vi "CCUP.vi"(3 "Device Category IN:":string(combo)="ATLAS18SS" caption="Device Category:", 4 "Batch No.:":string, 5 "Sensor Serial No.:":string, 6 "DB Serial No.:":string) -> (0 "Done!":bool)   [LabVIEW 2019]
doc: "Performs CV measurements according to ATLAS ITk Quality Control Specifications."
uses:
  general_VIs/globals/QC_RunInformation.vi
  general_VIs/globals/QC_MeasurementSetup.vi
  InstrControl/InstrumentSetup.vi
  InstrControl/Switching/Switching.lvclass
  InstrControl/SupplyControl/SupplyControl.lvclass
  InstrControl/LCRControl/LCRControl.lvclass
  InstrControl/ArduinoControl/ArduinoControl.lvclass
  <vilib>/Analysis/NI_AALBase.lvlib
  InstrControl/InstrControl.lvclass
panel:
  out "positive ramp?":bool
  out "Measured Capacitance [pF]":dbl
  in  "Continue":bool
  out "RH":dbl[](array[numeric]) caption="RH [%]" format="%#.2f"
  out "Temp.":dbl[](array[numeric]) caption="Temp. [°C]" format="%#.2f"
  in  "Measurement Configurations":bool
  in  "Frequency [Hz] Setup":i32=500 caption="Frequency [Hz]" format="%#.3p"
  in  "step interval [s] IN":i32=5 caption="step interval [s]"
  in  "step [V] IN":dbl=10.0 caption="step [V]" format="%.1f"
  in  "Final volts [V] IN":dbl=-500.0 caption="Final volts [V]"
  in  "Initial volts [V] IN":dbl caption="Initial volts [V]"
  in  "quit (no save)":bool
  in  "Quit & Save":bool
  out "Bias On/Off:":bool
  in  "Switching":string(combo)="Pickering Matrix"
  in  "Temperature":enum16{"Read Arduino", "Enter manually"}(ring)
  in  "LCR Meter":string(combo)="WayneKerr 6440B"
  in  "CV Supply":string(combo)="Keithley 2410"
  out "Initiated:":string
  in  "User:":string(combo)="Christoph"
  in  "Structure Name:":string
  # "Strip Sensor QC: Coupling Capacitance"
  # "DUT Description"
  # "Measurement Configuration"
  # "Hardware"
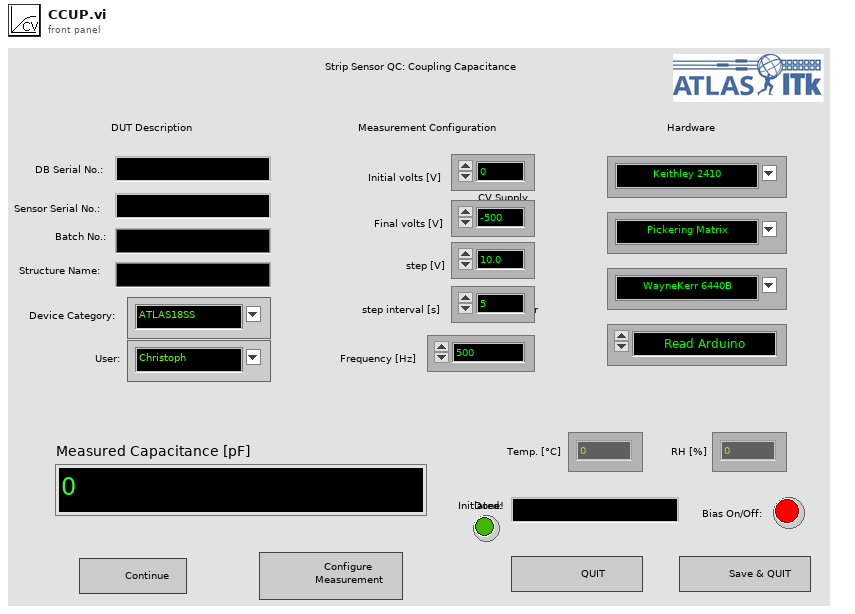
[diagram p1: front panel]
types:
  T1 = enum8{"Enabled", "Disabled", "Disabled and Grayed Out"}
  T2 = enum16{"Supply", "LCR", "Multimeter", "Switching"}
  T3 = enum16{"Reset", "Read Array", "Read Element", "Write Element", "Write Array", "Add Element", "Add Array"}
  T4 = enum16{"Reset", "Ground", "Striptest Bias", "Striptest SMU", "Striptest LCR", "IV", "CV", "Interstrip Cap", "Interstrip Res"}
  T5 = enum16{"Reset", "Ground", "Striptest Bias", "Striptest SMU", "Striptest LCR", "IV", "CV", "Interstrip Cap", "Interstrip Res", "PTP", "Implant Resistance", "Metal Resistance", "Coupling Capacitance"}
  T6 = cluster{"Supply":refnum<class "SupplyControl.lvclass">, "LCR":refnum<class "LCRControl.lvclass">, "Initial Voltage [V]":dbl, "Final Voltage [V]":dbl, "Step Size [V]":dbl, "Step Interval [s]":i32, "Number Of Steps":u32, "AC frequency [Hz]":i32, "RC Configuration":u16, "AC amplitude [V]":dbl, "Ramp down steps [V]":dbl, "Ramp down Interval [s]":i32, "Set Current Limit?":bool, "Current Limit [µA]":dbl, "Temperature Readout":enum16{"Read Arduino", "Enter manually"}, "Arduino":refnum<class "ArduinoControl.lvclass">, "Supply Name":string, "LCR Name":string, "V_depletion Limit [V]":dbl, "Switching":refnum<class "Switching.lvclass">, "Matrix used?":bool, "Matrix X Channels":cluster{"Bias Supply / SMU LO":i32, "Bias Supply / SMU HI":i32, "CV Box LO":i32, "CV Box HI":i32, "CV Box LO IN":i32, "CV Box HI IN":i32, "Volt meter LO":i32, "Volt meter HI":i32, "Mux1 C1":i32, "Mux1 C2":i32, "Mux2 C1":i32, "Mux2 C2":i32}, "Structure Name":string}
  T7 = cluster{"Sensor Serial No.:":string, "Wafer Serial No.:":string, "Batch:":string, "Manufacturer:":string, "Device Category:":string, "Database Serial No.:":string, "Date Initiated:":string, "Time Initiated:":string, "Test":string, "Instruments used:":string, "Probeplan used:":string, "End of Run comment:":string, "User:":string}
  T8 = cluster{"Institute":string, "Manufacturers":string[], "Devices":string[], "Serialnumbers Lookup DB":string, "Data directory":string, "Backup & screenshot directory":string, "List of known users":string[], "Measurement switch not used":bool, "Measurement Switch":string, "DUT Switch":string}
  T9 = cluster{"RC Configuration":u16, "AC amplitude [V]":dbl, "AC frequency [Hz]":i32, "WK6440B":refnum<class "WK6440B.lvclass">}
  T10 = cluster{"VISA address":refnum<visa-resource-name>, "T sensor":enum16{"SHT", "DS"}, "Arduino":refnum<class "ArduinoControl.lvclass">}
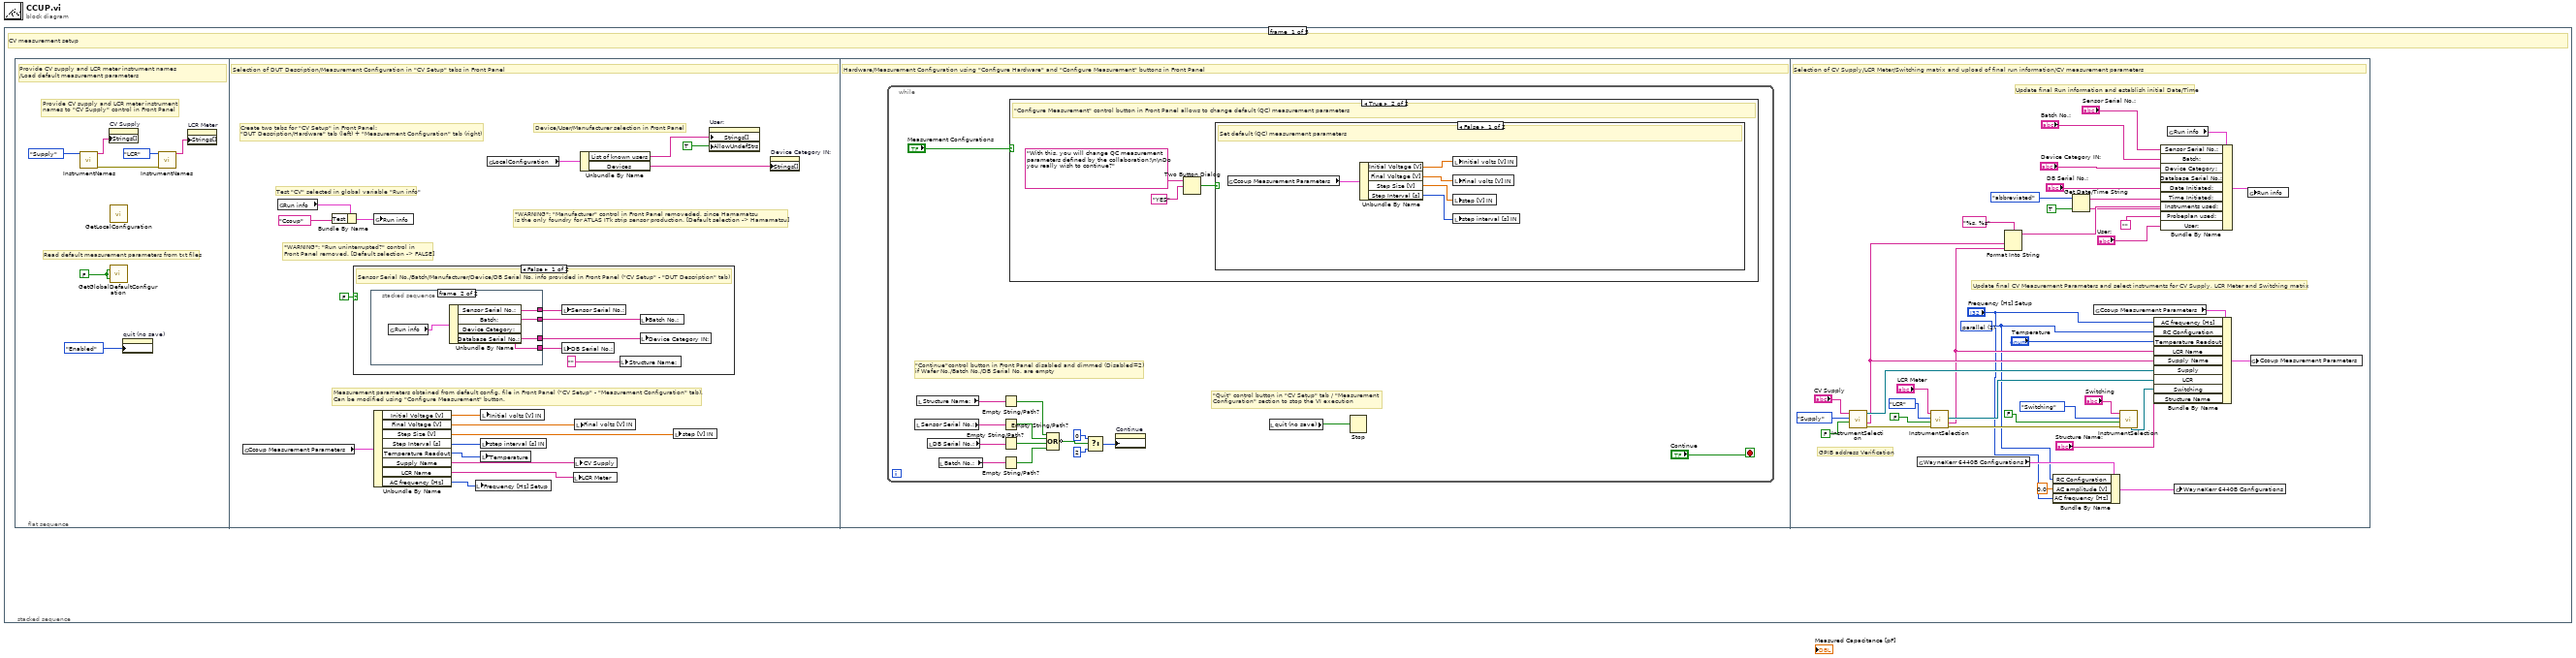
[diagram p0: block diagram]
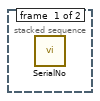
[diagram p2: hidden frame]
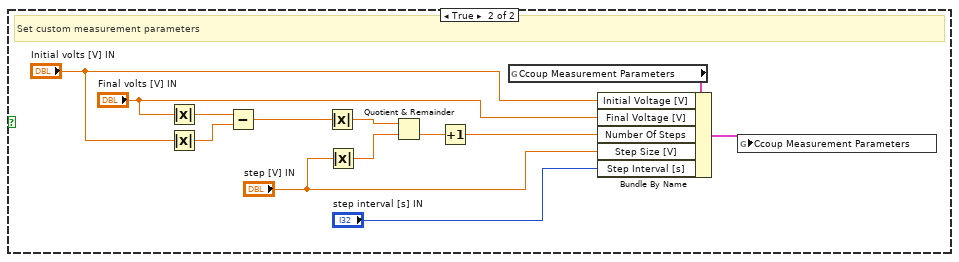
[diagram p5: hidden frame]
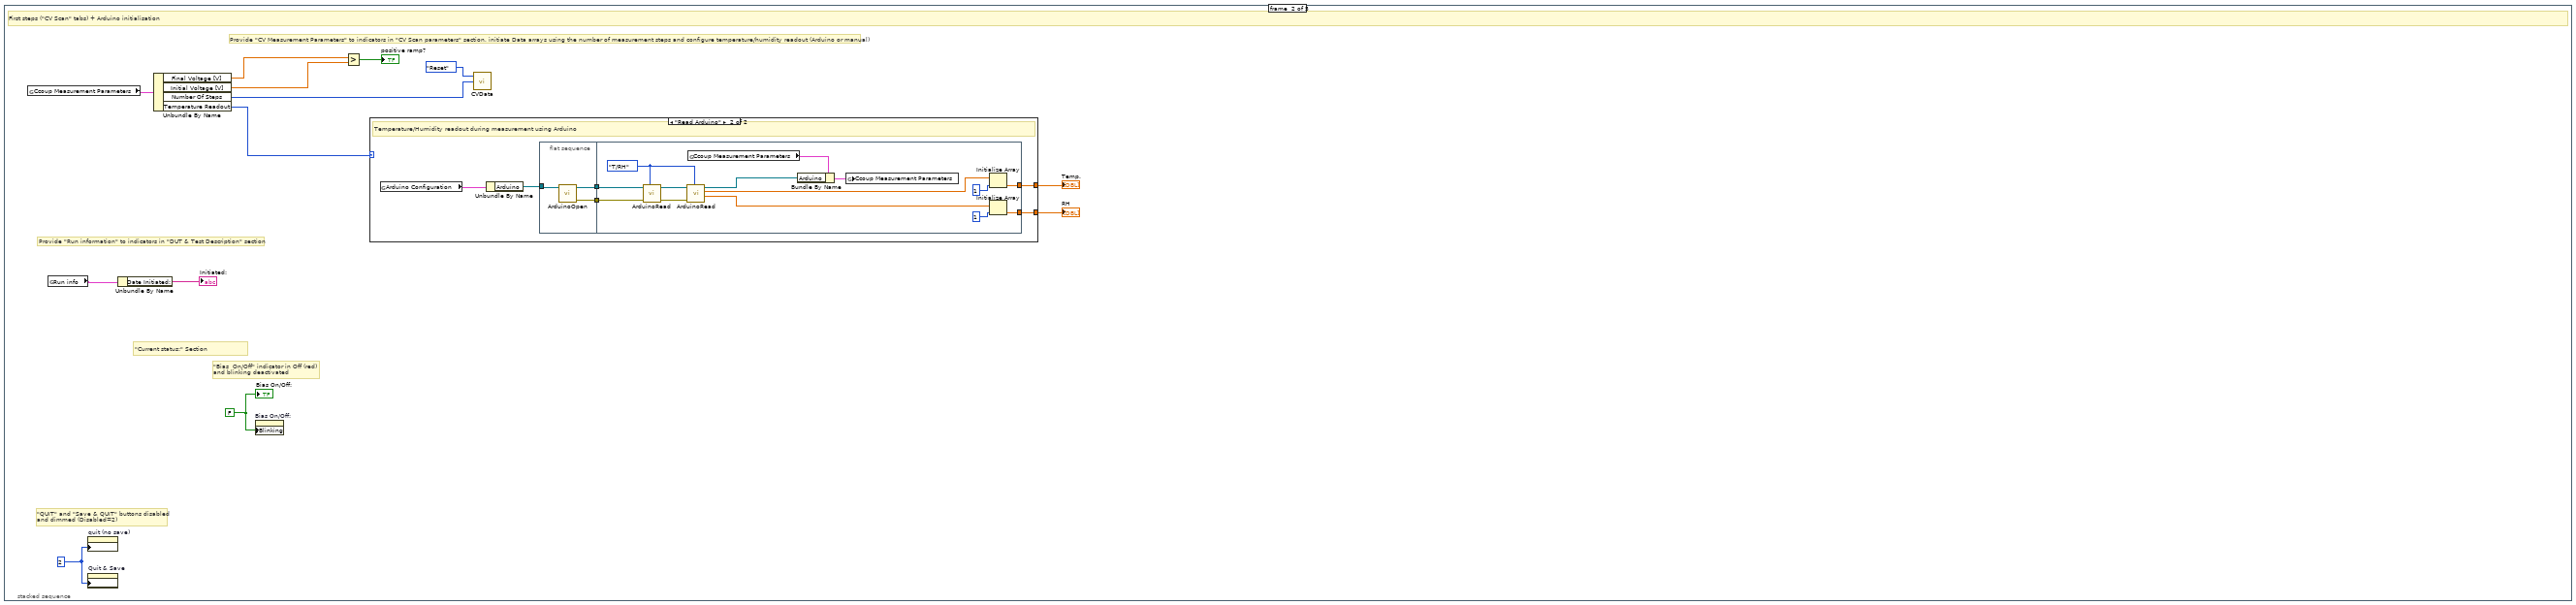
[diagram p6: hidden frame]
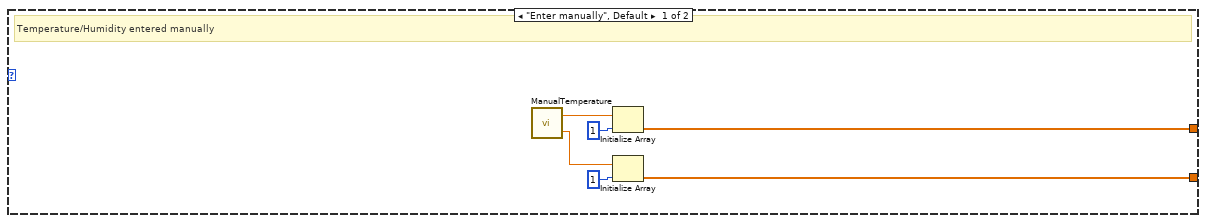
[diagram p7: hidden frame]
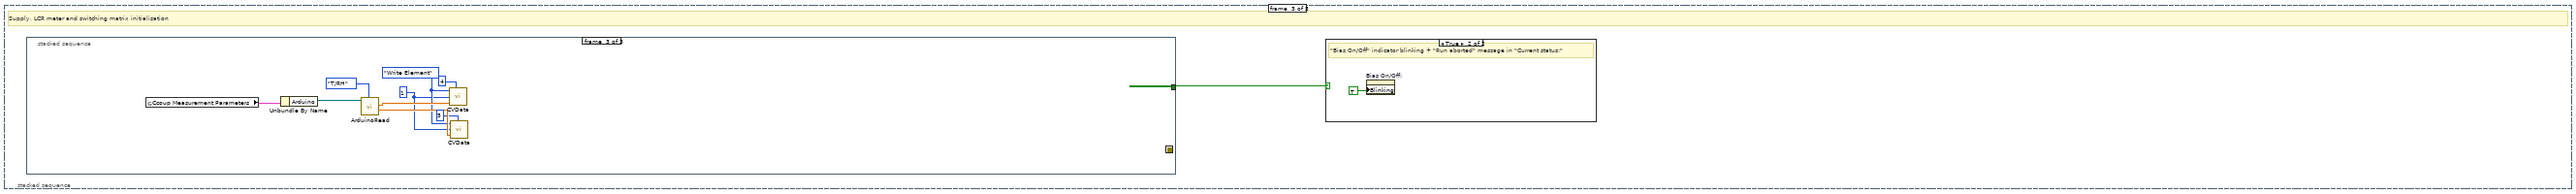
[diagram p8: hidden frame]
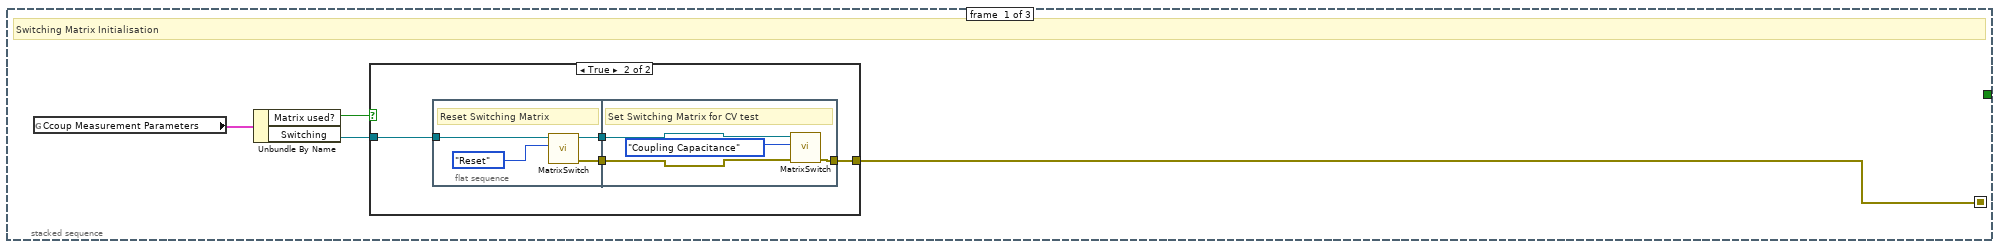
[diagram p9: hidden frame]
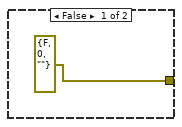
[diagram p10: hidden frame]
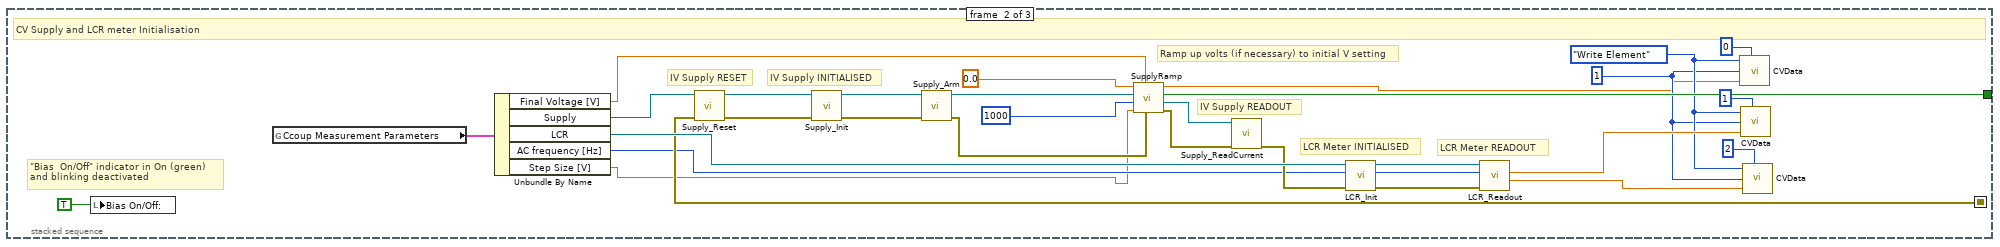
[diagram p11: hidden frame]
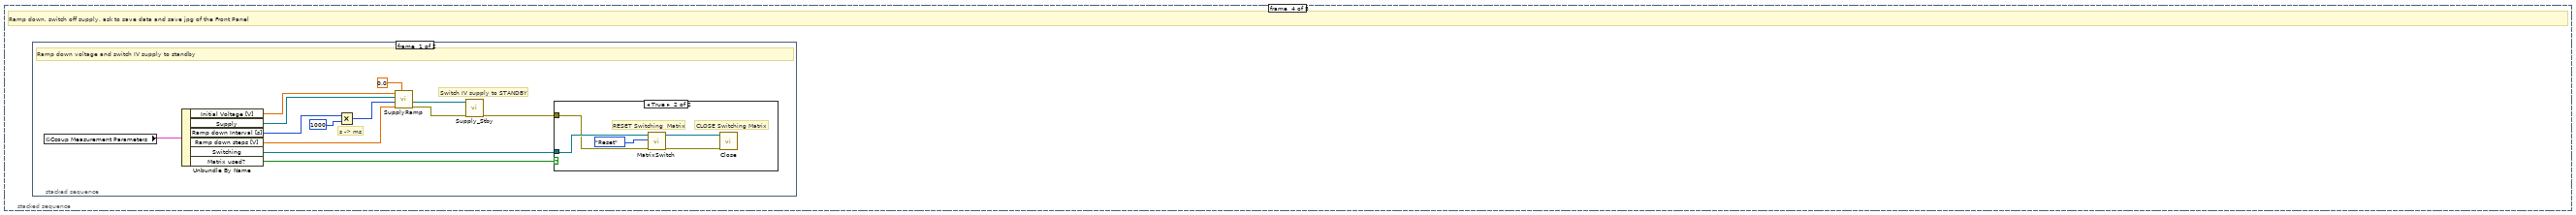
[diagram p13: hidden frame]
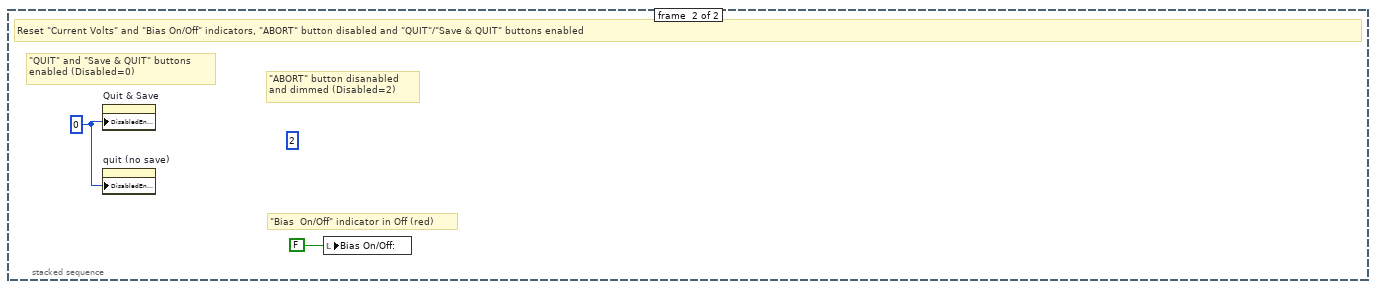
[diagram p15: hidden frame]
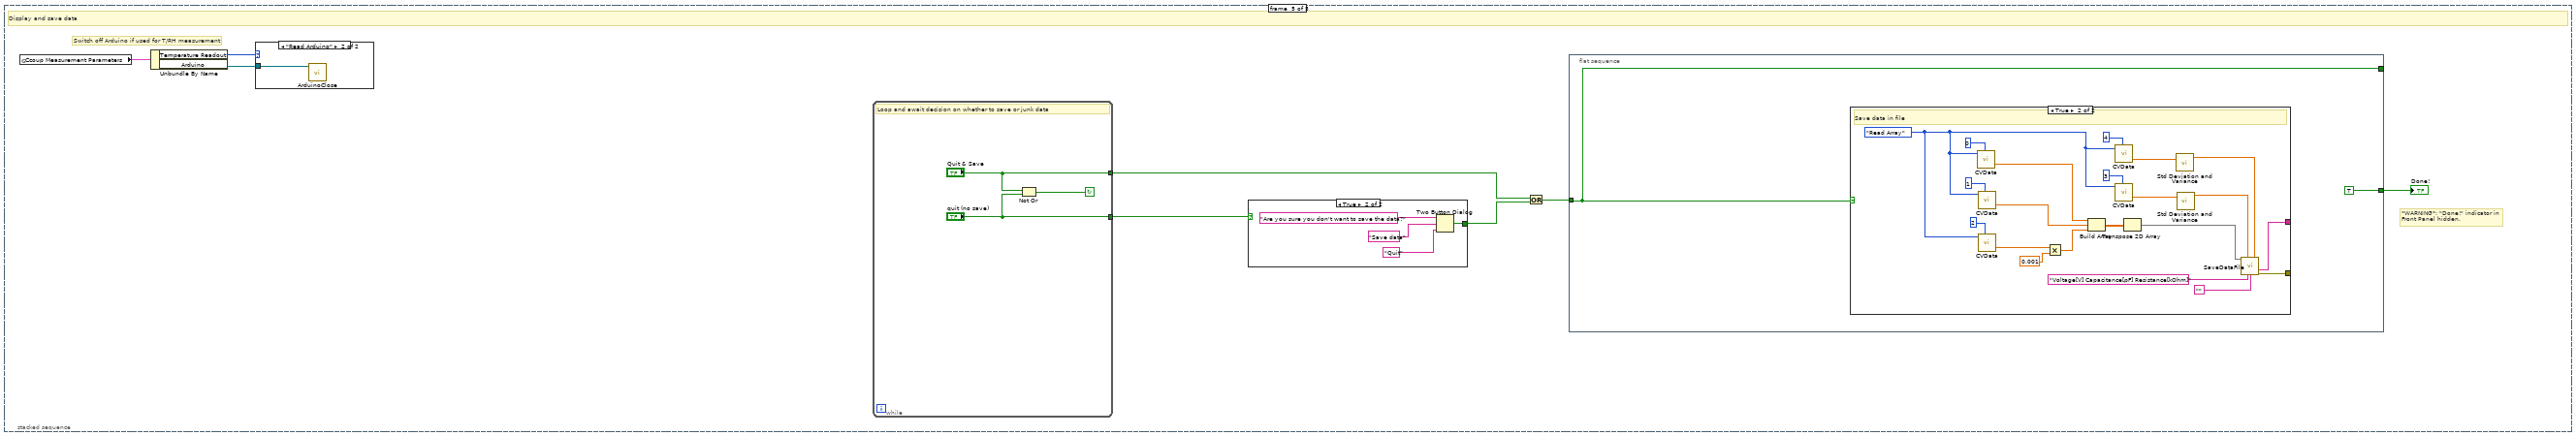
[diagram p16: hidden frame]
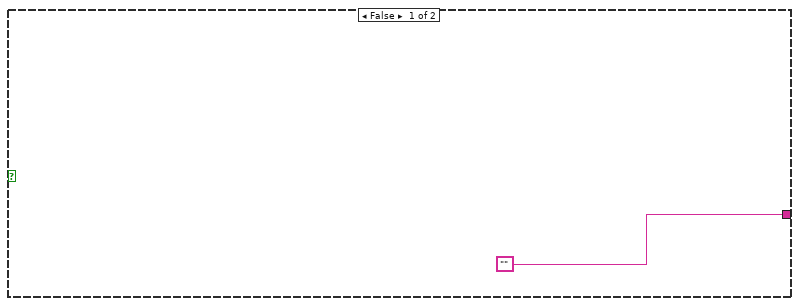
[diagram p17: hidden frame]
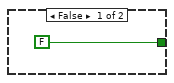
[diagram p19: hidden frame]
diagram:
  n1 = stacked-sequence {
    frame #0 {
      # "CV measurement setup"
      n2 = flat-sequence {
        frame #0 {
          w7 = FALSE
          # "Read default measurement parameters from txt files"
          # "Provide CV supply and LCR meter instrument \nnames to \"CV Supply\" control in Front Panel"
          # "Provide CV supply and LCR meter instrument names\n/Load default measurement parameters"
          n3 = call "InstrumentNames.vi"("Instrument type"=T2."Supply") -> ("error out"=w2:errorcluster, "Instrument names"=w4:string[])  [unwired: 9 in]
          n4 = property on="CV Supply" class="CmbBox"("Strings[]"=w4) -> ()  [unwired: 2 in, 2 out]
          n5 = call "GetGlobalDefaultConfiguration.vi"("DO NOT override instruments"=w7, "Read defaults?"=w7) -> ()  [unwired: 1 in, 1 out]
          n6 = call "GetLocalConfiguration.vi"() -> ()  [unwired: 3 in, 1 out]
          n7 = property on="quit (no save)" class="Bool (strict)"("DisabledEnum"=T1."Enabled" ("Disabled")) -> ()  [unwired: 2 in, 2 out]
          n8 = call "InstrumentNames.vi"("error in (no error)"=w2, "Instrument type"=T2."LCR") -> ("Instrument names"=w3:string[])  [unwired: 8 in, 1 out]
          n9 = property on="LCR Meter" class="CmbBox"("Strings[]"=w3) -> ()  [unwired: 2 in, 2 out]
        }
        frame #1 {
          # "Measurement parameters obtained from default config. file in Front Panel (\"CV Setup\" - \"Measurement Configuration\" tab).\nCan be modified using \"Configure Measurement\" button."
          # "*WARNING*: \"Run uninterrupted?\" control in \nFront Panel removed. [Default selection -> FALSE]"
          # "*WARNING*: \"Manufacturer\" control in Front Panel removeded, since Hamamatsu \nis the only foundry for ATLAS ITk strip sensor production. [Default selection -> Hamamatsu]"
          # "Test \"CV\" selected in global variable \"Run info\""
          # "Device/User/Manufacturer selection in Front Panel"
          # "Create two tabs for \"CV Setup\" in Front Panel:\n\"DUT Description/Hardware\" tab (left) + \"Measurement Configuration\" tab (right)"
          # "Selection of DUT Description/Measurement Configuration in \"CV Setup\" tabs in Front Panel"
          n10 = global read "QC_MeasurementSetup.vi" "Ccoup Measurement Parameters"() -> (w22:T6)
          n11 = global read "QC_RunInformation.vi" "Run info"() -> (w15:T7)
          n12 = Bundle By Name(cluster=w15, "Test"="Ccoup") -> (w16:T7)
          n13 = case shown="False" FALSE {
            frame False {
              # "Sensor Serial No./Batch/Manufacturer/Device/DB Serial No. info provided in Front Panel (\"CV Setup\" - \"DUT Description\" tab)"
              n14 = stacked-sequence {
                tunnel: [_ w34] -> w28
                tunnel: [_ w33] -> w27
                tunnel: [_ w32] -> w29
                tunnel: [_ w30] -> w26
                frame #0 {
                  n15 = call "SerialNo.vi"() -> ()  [unwired: 5 in, 1 out]
                }
                frame #1 {
                  n16 = global read "QC_RunInformation.vi" "Run info"() -> (w31:T7)
                  n17 = Unbundle By Name(w31) -> ("Sensor Serial No.:"=w34:string, "Batch:"=w33:string, "Device Category:"=w32:string, "Database Serial No.:"=w30:string)
                }
              }
              n18 = local write "Sensor Serial No.:"(w28) -> ()
              n19 = local write "DB Serial No.:"(w26) -> ()
              n20 = local write "Structure Name:"("" ("Structure Name:")) -> ()
              n21 = local write "Batch No.:"(w27) -> ()
              n22 = local write "Device Category IN:"(w29) -> ()
            }
            frame True {
            }
          }
          n23 = global write "QC_RunInformation.vi" "Run info"(w16) -> ()
          n24 = Unbundle By Name(w22) -> ("Initial Voltage [V]"=w11:dbl, "Final Voltage [V]"=w12:dbl, "Step Size [V]"=w13:dbl, "Step Interval [s]"=w14:i32, "Temperature Readout"=w24:enum16{"Read Arduino", "Enter manually"}, "Supply Name"=w23:string, "LCR Name"=w18:string, "AC frequency [Hz]"=w17:i32)
          n25 = local write "Frequency [Hz] Setup"(w17) -> ()
          n26 = local write "step interval [s] IN"(w14) -> ()
          n27 = local write "Temperature"(w24) -> ()
          n28 = local write "Initial volts [V] IN"(w11) -> ()
          n29 = global read "QC_RunInformation.vi" "LocalConfiguration"() -> (w21:T8)
          n30 = local write "LCR Meter"(w18) -> ()
          n31 = local write "CV Supply"(w23) -> ()
          n32 = local write "Final volts [V] IN"(w12) -> ()
          n33 = Unbundle By Name(w21) -> ("List of known users"=w20:string[], "Devices"=w10:string[])
          n34 = local write "step [V] IN"(w13) -> ()
          n35 = property on="User:" class="CmbBox"("Strings[]"=w20, "AllowUndefStrs"=TRUE) -> ()  [unwired: 2 in, 2 out]
          n36 = property on="Device Category IN:" class="CmbBox"("Strings[]"=w10) -> ()  [unwired: 2 in, 2 out]
        }
        frame #2 {
          # "Hardware/Measurement Configuration using \"Configure Hardware\" and \"Configure Measurement\" buttons in Front Panel"
          n37 = while {
            stop <- "Continue" stop-if-true
            # "\"Continue\"control button in Front Panel disabled and dimmed (Disabled=2) \nif Wafer No./Batch No./DB Serial No. are empty"
            # "\"Quit\" control button in \"CV Setup\" tab / \"Measurement \nConfiguration\" section to stop the VI execution"
            n38 = local read "Sensor Serial No.:"() -> (w49:string)
            n39 = local read "Structure Name:"() -> (w36:string)
            n40 = local read "DB Serial No.:"() -> (w48:string)
            n41 = local read "Batch No.:"() -> (w41:string)
            n42 = Empty String/Path?(string/path=w36) -> (empty?=w35:bool)
            n43 = Empty String/Path?(string/path=w49) -> (empty?=w46:bool)
            n44 = Empty String/Path?(string/path=w48) -> (empty?=w47:bool)
            n45 = Empty String/Path?(string/path=w41) -> (empty?=w40:bool)
            n46 = case shown="True" "Measurement Configurations" {
              frame False {
              }
              frame True {
                # "\"Configure Measurement\" control button in Front Panel allows to change default (QC) measurement parameters"
                n47 = Two Button Dialog(message="With this, you will change QC measurement parameters defined by the collaboration!\n\nDo you really wish to continue?", 2:"YES") -> (T button?=w50:bool)  [unwired: 1 in]
                n48 = case shown="False" w50 {
                  frame False {
                    # "Set default (QC) measurement parameters"
                    n49 = global read "QC_MeasurementSetup.vi" "Ccoup Measurement Parameters"() -> (w57:T6)
                    n50 = Unbundle By Name(w57) -> ("Initial Voltage [V]"=w54:dbl, "Final Voltage [V]"=w53:dbl, "Step Size [V]"=w55:dbl, "Step Interval [s]"=w56:i32)
                    n51 = local write "Initial volts [V] IN"(w54) -> ()
                    n52 = local write "Final volts [V] IN"(w53) -> ()
                    n53 = local write "step [V] IN"(w55) -> ()
                    n54 = local write "step interval [s] IN"(w56) -> ()
                  }
                  frame True {
                    # "Set custom measurement parameters"
                    n55 = Absolute Value(x="Final volts [V] IN") -> (abs(x)=w64:dbl)
                    n56 = Absolute Value(x="Initial volts [V] IN") -> (abs(x)=w65:dbl)
                    n57 = Subtract(x=w64, y=w65) -> (x-y=w68:dbl)
                    n58 = Absolute Value(x=w68) -> (abs(x)=w66:dbl)
                    n59 = Absolute Value(x="step [V] IN") -> (abs(x)=w67:dbl)
                    n60 = Quotient & Remainder(x=w66, y=w67) -> (floor(x/y)=w63:dbl)  [unwired: 1 out]
                    n61 = Increment(x=w63) -> (x+1=w59:dbl)
                    n62 = global read "QC_MeasurementSetup.vi" "Ccoup Measurement Parameters"() -> (w70:T6)
                    n63 = Bundle By Name(cluster=w70, "Initial Voltage [V]"="Initial volts [V] IN", "Final Voltage [V]"="Final volts [V] IN", "Number Of Steps"=w59, "Step Size [V]"="step [V] IN", "Step Interval [s]"="step interval [s] IN") -> (w69:T6)
                    n64 = global write "QC_MeasurementSetup.vi" "Ccoup Measurement Parameters"(w69) -> ()
                  }
                }
              }
            }
            n65 = Compound Arithmetic op=OR(w35, w46, w47, w40) -> (invert w45:bool)
            n66 = Select(t=0, s=w45, f=2) -> (s? t:f=w42:i32)
            n67 = property on="Continue" class="Bool"("DisabledEnum"=w42) -> ()  [unwired: 2 in, 2 out]
            n68 = local read "quit (no save)"() -> (w38:bool)
            n69 = Stop(stop? (T)=w38) -> ()
          }
        }
        frame #3 {
          w72 = u16 1 items=["serial", "parallel"] ("RC Configuration")
          # "Update final Run information and establish initial Date/Time"
          # "Update final CV Measurement Parameters and select instruments for CV Supply, LCR Meter and Switching matrix"
          # "GPIB address Verification"
          # "Selection of CV Supply/LCR Meter/Switching matrix and upload of final run information/CV measurement parameters"
          n70 = call "InstrumentSelection.vi"("Verify GPIB address"=FALSE, "Instrument type"=T2."Supply", "Instrument name IN"="CV Supply") -> ("error out"=w95:errorcluster, "Instrument name OUT"=w78:string, "Supply"=w94:refnum<class "SupplyControl.lvclass">)  [unwired: 3 in, 3 out]
          n71 = global read "InstrumentSetup.vi" "WayneKerr 6440B Configurations"() -> (w74:T9)
          n72 = call "InstrumentSelection.vi"("error in (no error)"=w95, "Verify GPIB address"=FALSE, "Instrument type"=T2."LCR", "Instrument name IN"="LCR Meter") -> ("error out"=w91:errorcluster, "Instrument name OUT"=w77:string, "LCR"=w93:refnum<class "LCRControl.lvclass">)  [unwired: 2 in, 3 out]
          n73 = Format Into String(format string="%s, %s", w78, w77) -> (resulting string=w98:string)  [unwired: 2 in, 1 out]
          n74 = Bundle By Name(cluster=w74, "RC Configuration"=w72, "AC amplitude [V]"=0.0, "AC frequency [Hz]"="Frequency [Hz] Setup") -> (w75:T9)
          n75 = Get Date/Time String(date format (0)=enum16{"short", "long", "abbreviated"}."abbreviated", want seconds? (F)=TRUE) -> (date string=w86:string, time string=w85:string)  [unwired: 1 in]
          n76 = global read "QC_MeasurementSetup.vi" "Ccoup Measurement Parameters"() -> (w108:T6)
          n77 = call "InstrumentSelection.vi"("error in (no error)"=w91, "Verify GPIB address"=FALSE, "Instrument type"=T2."Switching", "Instrument name IN"="Switching") -> ("Switching"=w90:refnum<class "Switching.lvclass">)  [unwired: 2 in, 5 out]
          n78 = Bundle By Name(cluster=w108, "AC frequency [Hz]"="Frequency [Hz] Setup", "RC Configuration"=w72, "Temperature Readout"="Temperature", "LCR Name"=w77, "Supply Name"=w78, "Supply"=w94, "LCR"=w93, "Switching"=w90, "Structure Name"="Structure Name:") -> (w109:T6)
          n79 = global read "QC_RunInformation.vi" "Run info"() -> (w105:T7)
          n80 = Bundle By Name(cluster=w105, "Sensor Serial No.:"="Sensor Serial No.:", "Batch:"="Batch No.:", "Device Category:"="Device Category IN:", "Database Serial No.:"="DB Serial No.:", "Date Initiated:"=w86, "Time Initiated:"=w85, "Instruments used:"=w98, "Probeplan used:"="", "User:"="User:") -> (w104:T7)
          n81 = global write "InstrumentSetup.vi" "WayneKerr 6440B Configurations"(w75) -> ()
          n82 = global write "QC_RunInformation.vi" "Run info"(w104) -> ()
          n83 = global write "QC_MeasurementSetup.vi" "Ccoup Measurement Parameters"(w109) -> ()
        }
      }
    }
    frame #1 {
      w118 = 2
      w117 = FALSE ("Visible")
      # "Provide \"CV Measurement Parameters\" to indicators in \"CV Scan parameters\" section, initiate Data arrays using the number of measurement steps and configure temperature/humidity readout (Arduino or manual)"
      # "\"Current status:\" Section"
      # "Provide \"Run information\" to indicators in \"DUT & Test Description\" section"
      # "\"Bias  On/Off\" indicator in Off (red)\nand blinking deactivated"
      # "\"QUIT\" and \"Save & QUIT\" buttons disabled\nand dimmed (Disabled=2)"
      # "First steps (\"CV Scan\" tabs) + Arduino initialisation"
      n84 = global read "QC_MeasurementSetup.vi" "Ccoup Measurement Parameters"() -> (w113:T6)
      n85 = global read "QC_RunInformation.vi" "Run info"() -> (w122:T7)
      n86 = property on="quit (no save)" class="Bool (strict)"("DisabledEnum"=w118) -> ()  [unwired: 2 in, 2 out]
      n87 = property on="Quit & Save" class="Bool"("DisabledEnum"=w118) -> ()  [unwired: 2 in, 2 out]
      n88 = Unbundle By Name(w122) -> ("Date Initiated:"=→"Initiated:":string)
      n89 = Unbundle By Name(w113) -> ("Final Voltage [V]"=w110:dbl, "Initial Voltage [V]"=w111:dbl, "Number Of Steps"=w121:u32, "Temperature Readout"=w119:enum16{"Read Arduino", "Enter manually"})
      n90 = property on="Bias On/Off:" class="Bool (strict)"("Blinking"=w117) -> ()  [unwired: 2 in, 2 out]
      n91 = Greater?(x=w110, y=w111) -> (0:→"positive ramp?":bool)
      n92 = case shown="\"Read Arduino\"" w119 {
        tunnel: [w127 w134] -> w120
        tunnel: [w124 w133] -> w114
        frame "Enter manually", Default {
          # "Temperature/Humidity entered manually"
          n93 = call "ManualTemperature.vi"() -> ("Humidity [%] out"=w123:dbl, "Temperature [°C] out"=w128:dbl)
          n94 = Initialize Array(w128, 1) -> (w127:dbl[])
          n95 = Initialize Array(w123, 1) -> (w124:dbl[])
        }
        frame "Read Arduino" {
          # "Temperature/Humidity readout during measurement using Arduino"
          n96 = global read "InstrumentSetup.vi" "Arduino Configuration"() -> (w130:T10)
          n97 = Unbundle By Name(w130) -> ("Arduino"=w129:refnum<class "ArduinoControl.lvclass">)
          n98 = flat-sequence {
            tunnel: [w135] -> w132
            tunnel: [w137] -> w131
            tunnel: w129 -> [w136]
            tunnel: [w151] -> w134
            tunnel: [w148] -> w133
            tunnel: w132 -> [w140]
            tunnel: w131 -> [w141]
            frame #0 {
              n99 = call "ArduinoOpen.vi"("ArduinoControl in"=w136) -> ("error out"=w137:errorcluster, "ArduinoControl out"=w135:refnum<class "ArduinoControl.lvclass">)  [unwired: 9 in]
            }
            frame #1 {
              w142 = enum16{"T/RH", "Interlock", "Edgesense"}."T/RH" ("Arduino function")
              n100 = call "ArduinoRead.vi"("Arduino function"=w142, "error in (no error)"=w141, "ArduinoControl in"=w140) -> ("error out"=w138:errorcluster, "ArduinoControl out"=w139:refnum<class "ArduinoControl.lvclass">)  [unwired: 3 in, 4 out]
              n101 = call "ArduinoRead.vi"("Arduino function"=w142, "error in (no error)"=w138, "ArduinoControl in"=w139) -> ("rel. Humidity [%]"=w146:dbl, "Temperature [°C]"=w147:dbl, "ArduinoControl out"=w145:refnum<class "ArduinoControl.lvclass">)  [unwired: 3 in, 3 out]
              n102 = global read "QC_MeasurementSetup.vi" "Ccoup Measurement Parameters"() -> (w144:T6)
              n103 = Bundle By Name(cluster=w144, "Arduino"=w145) -> (w143:T6)
              n104 = global write "QC_MeasurementSetup.vi" "Ccoup Measurement Parameters"(w143) -> ()
              n105 = Initialize Array(w147, 1) -> (w151:dbl[])
              n106 = Initialize Array(w146, 1) -> (w148:dbl[])
            }
          }
        }
      }
      "Temp." <- w120
      "RH" <- w114
      n107 = call "CVData.vi"("Action"=T3."Reset", "Array Size / Index"=w121) -> ()  [unwired: 3 in, 2 out]
      "Bias On/Off:" <- w117
    }
    frame #2 {
      # "Supply, LCR meter and switching matrix initialisation"
      n108 = stacked-sequence {
        seq-local: [w154 _ _] -> [_ w183 _]
        tunnel: [_ w187 _] -> w152
        frame #0 {
          # "Switching Matrix Initialisation"
          n109 = global read "QC_MeasurementSetup.vi" "Ccoup Measurement Parameters"() -> (w153:T6)
          n110 = Unbundle By Name(w153) -> ("Matrix used?"=w156:bool, "Switching"=w155:refnum<class "Switching.lvclass">)
          n111 = case shown="True" w156 {
            tunnel: w155 -> [_ w158]
            tunnel: [errorcluster {"status"=FALSE, "code"=0, "source"=""} ("error constant") w159] -> w154
            frame False {
            }
            frame True {
              n112 = flat-sequence {
                tunnel: [w165] -> w161
                tunnel: [w164] -> w160
                tunnel: w158 -> [w163]
                tunnel: w161 -> [w169]
                tunnel: w160 -> [w168]
                tunnel: [w167] -> w159
                frame #0 {
                  # "Reset Switching Matrix"
                  n113 = call-dynamic "MatrixSwitch.vi"("Action"=T4."Reset", "Switching in"=w163) -> ("error out"=w165:errorcluster, "Switching out"=w164:refnum<class "Switching.lvclass">)  [unwired: 7 in, 1 out]
                }
                frame #1 {
                  # "Set Switching Matrix for CV test"
                  n114 = call-dynamic "MatrixSwitch.vi"("error in (no error)"=w169, "Action"=T5."Coupling Capacitance", "Switching in"=w168) -> ("error out"=w167:errorcluster)  [unwired: 6 in, 2 out]
                }
              }
            }
          }
        }
        frame #1 {
          w175 = u32 1 ("Array Size / Index")
          w176 = T3."Write Element" ("Action")
          # "IV Supply READOUT"
          # "LCR Meter READOUT"
          # "LCR Meter INITIALISED"
          # "IV Supply INITIALISED"
          # "IV Supply RESET"
          # "\"Bias  On/Off\" indicator in On (green)\nand blinking deactivated"
          # "Ramp up volts (if necessary) to initial V setting"
          # "CV Supply and LCR meter Initialisation"
          n115 = local write "Bias On/Off:"(TRUE ("Compliance?")) -> ()
          n116 = global read "QC_MeasurementSetup.vi" "Ccoup Measurement Parameters"() -> (w195:T6)
          n117 = Unbundle By Name(w195) -> ("Final Voltage [V]"=w179:dbl, "Supply"=w193:refnum<class "SupplyControl.lvclass">, "LCR"=w192:refnum<class "LCRControl.lvclass">, "AC frequency [Hz]"=w180:i32, "Step Size [V]"=w178:dbl)
          n118 = call-dynamic "Supply_Reset.vi"("error in (no error)"=w183, "SupplyControl in"=w193) -> ("error out"=w197:errorcluster, "SupplyControl out"=w199:refnum<class "SupplyControl.lvclass">)  [unwired: 8 in]
          n119 = call-dynamic "Supply_Init.vi"("error in (no error)"=w197, "SupplyControl in"=w199) -> ("error out"=w196:errorcluster, "SupplyControl out"=w198:refnum<class "SupplyControl.lvclass">)  [unwired: 8 in]
          n120 = call-dynamic "Supply_Arm.vi"("error in (no error)"=w196, "SupplyControl in"=w198) -> ("error out"=w185:errorcluster, "SupplyControl out"=w186:refnum<class "SupplyControl.lvclass">)  [unwired: 8 in]
          n121 = call "SupplyRamp.vi"("error in"=w185, "Requested Voltage"=w179, "Step Size"=w178, "Step Delay"=1000, "Supply IN"=w186, "Starting Voltage"=0.0) -> ("error out"=w188:errorcluster, "Supply OUT"=w189:refnum<class "SupplyControl.lvclass">, "Compliance exceeded"=w187:bool, "Current Voltage"=w170:dbl)  [unwired: 2 in]
          n122 = call-dynamic "Supply_ReadCurrent.vi"("error in (no error)"=w188, "SupplyControl in"=w189) -> ("error out"=w184:errorcluster)  [unwired: 7 in, 2 out]
          n123 = call-dynamic "LCR_Init.vi"("error in (no error)"=w184, "LCRControl in"=w192) -> ("error out"=w181:errorcluster, "LCRControl out"=w182:refnum<class "LCRControl.lvclass">)  [unwired: 8 in]
          n124 = call-dynamic "LCR_Readout.vi"("error in (no error)"=w181, "Frequency in Hz"=w180, "LCRControl in"=w182) -> ("Resistance in Ohm"=w174:dbl, "Capacitance in pF"=w177:dbl)  [unwired: 5 in, 2 out]
          n125 = call "CVData.vi"("Action"=w176, "Array No."=u32 0, "Array Size / Index"=w175, "Data IN"=w170) -> ()  [unwired: 1 in, 2 out]
          n126 = call "CVData.vi"("Action"=w176, "Array No."=u32 1, "Array Size / Index"=w175, "Data IN"=w177) -> ()  [unwired: 1 in, 2 out]
          n127 = call "CVData.vi"("Action"=w176, "Array No."=u32 2, "Array Size / Index"=w175, "Data IN"=w174) -> ()  [unwired: 1 in, 2 out]
        }
        frame #2 {
          w202 = u32 1 ("Array Size / Index")
          w203 = T3."Write Element" ("Action")
          n128 = global read "QC_MeasurementSetup.vi" "Ccoup Measurement Parameters"() -> (w208:T6)
          n129 = Unbundle By Name(w208) -> ("Arduino"=w207:refnum<class "ArduinoControl.lvclass">)
          n130 = call "ArduinoRead.vi"("Arduino function"=enum16{"T/RH", "Interlock", "Edgesense"}."T/RH", "ArduinoControl in"=w207) -> ("rel. Humidity [%]"=w204:dbl, "Temperature [°C]"=w205:dbl)  [unwired: 4 in, 4 out]
          n131 = call "CVData.vi"("Action"=w203, "Array No."=u32 4, "Array Size / Index"=w202, "Data IN"=w205) -> ()  [unwired: 1 in, 2 out]
          n132 = call "CVData.vi"("Action"=w203, "Array No."=u32 5, "Array Size / Index"=w202, "Data IN"=w204) -> ()  [unwired: 1 in, 2 out]
        }
      }
      n133 = case shown="True" w152 {
        frame False {
        }
        frame True {
          # "\"Bias On/Off\" indicator blinking + \"Run aborted\" message in \"Current status:\""
          n134 = property on="Bias On/Off:" class="Bool (strict)"("Blinking"=TRUE) -> ()  [unwired: 2 in, 2 out]
        }
      }
    }
    frame #3 {
      # "Ramp down, switch off supply, ask to save data and save jpg of the Front Panel"
      n135 = stacked-sequence {
        frame #0 {
          # "Switch IV supply to STANDBY"
          # "s -> ms"
          # "Ramp down voltage and switch IV supply to standby"
          n136 = global read "QC_MeasurementSetup.vi" "Ccoup Measurement Parameters"() -> (w219:T6)
          n137 = Unbundle By Name(w219) -> ("Initial Voltage [V]"=w210:dbl, "Supply"=w218:refnum<class "SupplyControl.lvclass">, "Ramp down Interval [s]"=w212:i32, "Ramp down steps [V]"=w211:dbl, "Switching"=w214:refnum<class "Switching.lvclass">, "Matrix used?"=w213:bool)
          n138 = Multiply(x=w212, y=1000) -> (x*y=w221:i32)
          n139 = call "SupplyRamp.vi"("Requested Voltage"=0.0, "Step Size"=w211, "Step Delay"=w221, "Supply IN"=w218, "Starting Voltage"=w210) -> ("error out"=w216:errorcluster, "Supply OUT"=w217:refnum<class "SupplyControl.lvclass">)  [unwired: 3 in, 2 out]
          n140 = call-dynamic "Supply_Stby.vi"("error in (no error)"=w216, "SupplyControl in"=w217) -> ("error out"=w215:errorcluster)  [unwired: 8 in, 1 out]
          n141 = case shown="True" w213 {
            tunnel: w214 -> [_ w227]
            tunnel: w215 -> [_ w226]
            frame False {
            }
            frame True {
              # "CLOSE Switching Matrix"
              # "RESET Switching  Matrix"
              n142 = call-dynamic "MatrixSwitch.vi"("error in (no error)"=w226, "Action"=T4."Reset", "Switching in"=w227) -> ("error out"=w223:errorcluster, "Switching out"=w224:refnum<class "Switching.lvclass">)  [unwired: 6 in, 1 out]
              n143 = call-dynamic "Close.vi"("error in (no error)"=w223, "Switching in"=w224) -> ()  [unwired: 8 in, 2 out]
            }
          }
        }
        frame #1 {
          (unwired) 2
          w229 = 0
          # "\"QUIT\" and \"Save & QUIT\" buttons \nenabled (Disabled=0)"
          # "\"ABORT\" button disanabled \nand dimmed (Disabled=2)"
          # "\"Bias  On/Off\" indicator in Off (red)"
          # "Reset \"Current Volts\" and \"Bias On/Off\" indicators, \"ABORT\" button disabled and \"QUIT\"/\"Save & QUIT\" buttons enabled"
          n144 = property on="Quit & Save" class="Bool"("DisabledEnum"=w229) -> ()  [unwired: 2 in, 2 out]
          n145 = property on="quit (no save)" class="Bool (strict)"("DisabledEnum"=w229) -> ()  [unwired: 2 in, 2 out]
          n146 = local write "Bias On/Off:"(FALSE ("Visible")) -> ()
        }
      }
    }
    frame #4 {
      # "*WARNING*: \"Done!\" indicator in \nFront Panel hidden."
      # "Switch off Arduino if used for T/RH measurement"
      # "Display and save data"
      n147 = global read "QC_MeasurementSetup.vi" "Ccoup Measurement Parameters"() -> (w234:T6)
      n148 = Unbundle By Name(w234) -> ("Temperature Readout"=w233:enum16{"Read Arduino", "Enter manually"}, "Arduino"=w231:refnum<class "ArduinoControl.lvclass">)
      n149 = case shown="\"Read Arduino\"" w233 {
        tunnel: w231 -> [_ w262]
        frame "Enter manually", Default {
        }
        frame "Read Arduino" {
          n150 = call "ArduinoClose.vi"("ArduinoControl in"=w262) -> ()  [unwired: 9 in, 2 out]
        }
      }
      n151 = while {
        tunnel: ["Quit & Save"] -> w236
        tunnel: ["quit (no save)"] -> w235
        stop <- w264 continue-if-true
        # "Loop and await decision on whether to save or junk data"
        n152 = Not Or(1:"quit (no save)", 2:"Quit & Save") -> (0:w264:bool)
      }
      n153 = case shown="True" w235 {
        tunnel: [FALSE w267] -> w237
        frame False {
        }
        frame True {
          n154 = Two Button Dialog(message="Are you sure you don't want to save the data?", 1:"Quit" ("F button name (\"Cancel\")"), 2:"Save data" ("T button name (\"OK\")")) -> (T button?=w267:bool)
        }
      }
      n155 = Or(x=w236, y=w237) -> (x .or. y?=w232:bool)
      n156 = flat-sequence {
        tunnel: w232 -> [w238]
        tunnel: [w238] -> _
        tunnel: [TRUE] -> w230
        frame #0 {
          n157 = case shown="True" w238 {
            tunnel: ["" w261] -> _
            tunnel: [_ w247] -> _
            frame False {
            }
            frame True {
              w245 = T3."Read Array" ("Action")
              # "Save data in file"
              n158 = call "CVData.vi"("Action"=w245, "Array No."=u32 0 ("Action")) -> ("Array OUT"=w253:dbl[])  [unwired: 3 in, 1 out]
              n159 = call "CVData.vi"("Action"=w245, "Array No."=u32 1 ("Action")) -> ("Array OUT"=w252:dbl[])  [unwired: 3 in, 1 out]
              n160 = call "CVData.vi"("Action"=w245, "Array No."=u32 2 ("Action")) -> ("Array OUT"=w243:dbl[])  [unwired: 3 in, 1 out]
              n161 = Multiply(x=w243, y=0.001) -> (x*y=w242:dbl[])
              n162 = Build Array(w253, w252, w242) -> (w251:dbl[][])
              n163 = call "CVData.vi"("Action"=w245, "Array No."=u32 4 ("Action")) -> ("Array OUT"=w259:dbl[])  [unwired: 3 in, 1 out]
              n164 = call "CVData.vi"("Action"=w245, "Array No."=u32 3 ("Action")) -> ("Array OUT"=w258:dbl[])  [unwired: 3 in, 1 out]
              n165 = Transpose 2D Array(2D array=w251) -> (transposed array=w250:dbl[][])
              n166 = call <vilib>:"Std Deviation and Variance.vi"("X"=w259) -> ("mean"=w248:dbl)  [unwired: 1 in, 2 out]
              n167 = call <vilib>:"Std Deviation and Variance.vi"("X"=w258) -> ("mean"=w249:dbl)  [unwired: 1 in, 2 out]
              n168 = call "SaveDataFile.vi"("Data Array"=w250, "Temperature"=w249, "Humidity"=w248, "Array Titles"="Voltage[V] Capacitance[pF] Resistance[kOhm]", "Strip Segment"="") -> ("Path + Filename OUT"=w261:string, "Error Out"=w247:errorcluster)  [unwired: 7 in, 2 out]
            }
          }
        }
      }
      "Done!" <- w230
    }
  }
